vi "FacadeResizable1DArray(I32).vi"(0 "Data In":T4, 2 "Display State In":T2, 3 "Container State":T3) -> (6 "Data Out":T4, 7 "Display State Out":T2, 8 "Action":T1)   [LabVIEW 2011, in "Resizable1DArray(I32).xctl"]
uses:
  <vilib>/_probes/SAPHIR/ViBox - Probes/Resizable1DArray/Resizable1DArray(I32)/Resizable1DArray(I32).xctl
  <vilib>/_probes/SAPHIR/ViBox - Probes/Resizable1DArray/Resizable1DArray(I32)/DataResizable1DArray(I32).ctl
  <vilib>/_xctls/Container State.ctl
  <vilib>/_probes/SAPHIR/ViBox - Probes/Resizable1DArray/Resizable1DArray(I32)/StateResizable1DArray(I32).ctl
  <vilib>/_xctls/Action.ctl
  <vilib>/_xctls/XControlSupport.lvlib
panel:
  in  "Format":string caption="Format :"
  out "Numeric":i32
  out "[I32]":i32[](array[numeric])
  # "Display Options"
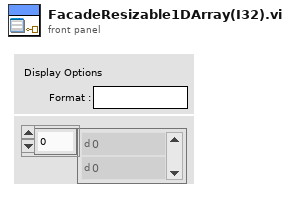
[diagram p1: front panel]
types:
  T1 = typedef "XControlSupport.lvlib/Action.ctl" = cluster{"Data Changed?":bool, "State Changed?":bool, "Action Name":string}
  T2 = typedef "Resizable1DArray(I32).xctl/StateResizable1DArray(I32).ctl" = cluster{"Height":u32}
  T3 = typedef "XControlSupport.lvlib/Container State.ctl" = cluster{"Indicator?":bool, "Run Mode?":bool, " Refnum":refnum<vi>}
  T4 = typedef "Resizable1DArray(I32).xctl/DataResizable1DArray(I32).ctl" = i32[]
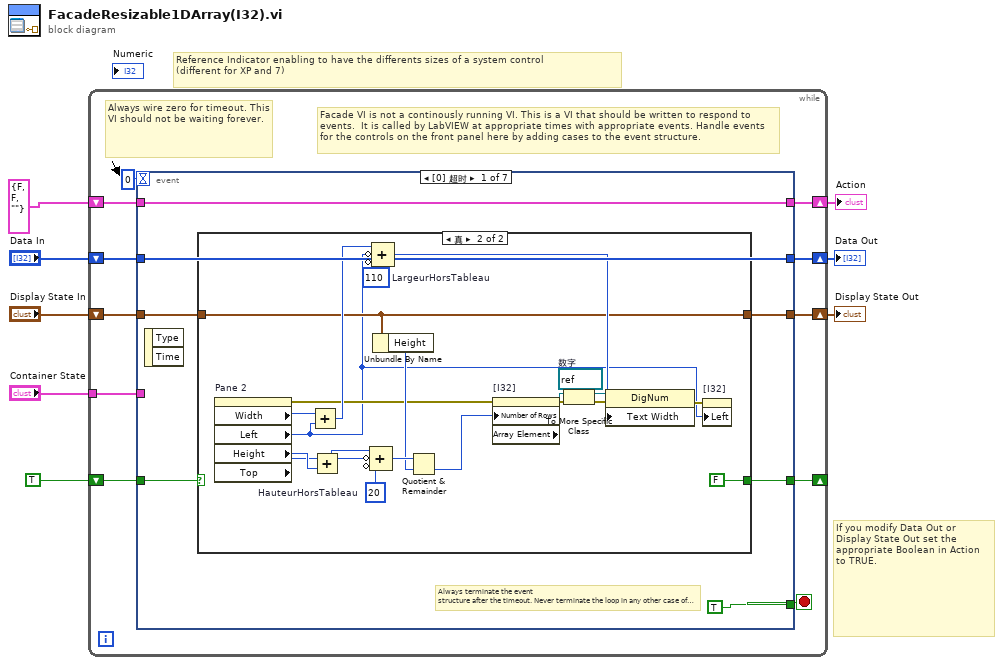
[diagram p0: block diagram]
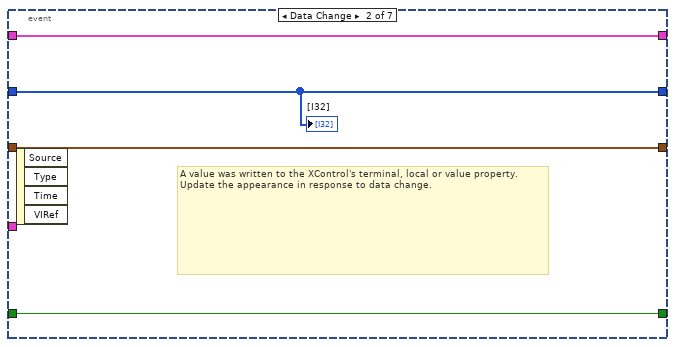
[diagram p3: hidden frame]
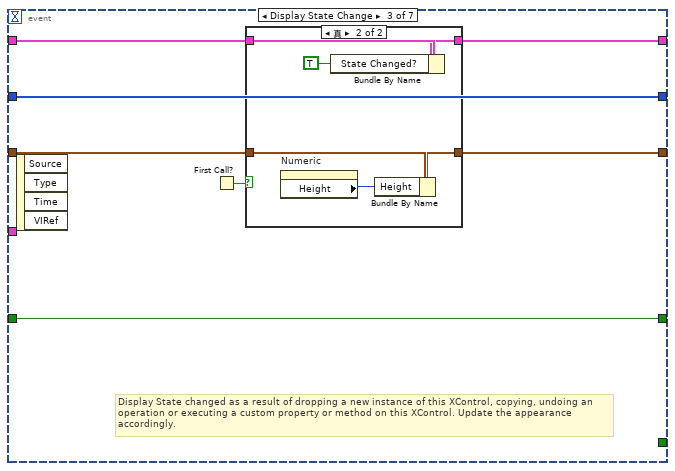
[diagram p4: hidden frame]
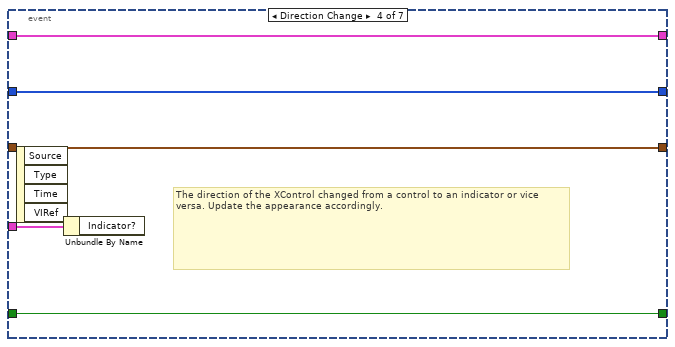
[diagram p6: hidden frame]
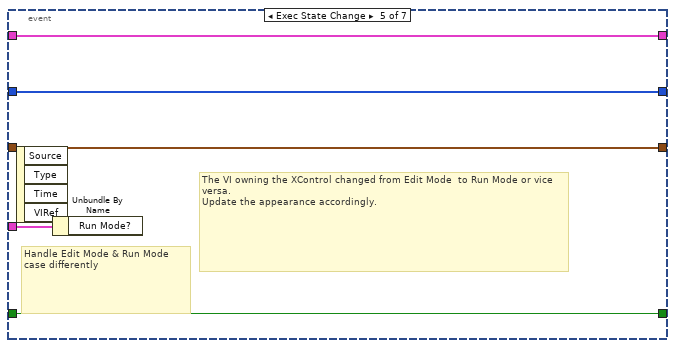
[diagram p7: hidden frame]
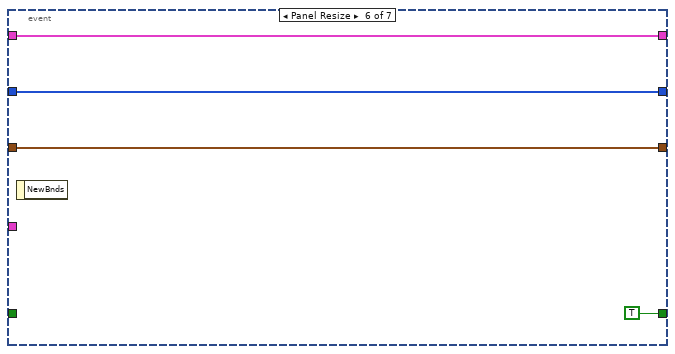
[diagram p8: hidden frame]
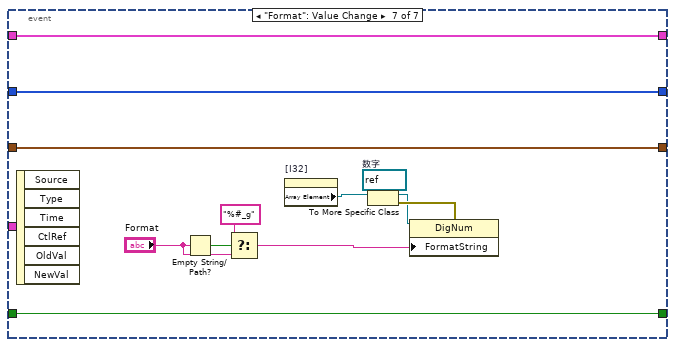
[diagram p9: hidden frame]
diagram:
  # "Reference Indicator enabling to have the differents sizes of a system control\n(different for XP and 7)"
  # "If you modify Data Out or\nDisplay State Out set the\nappropriate Boolean in Action\nto TRUE."
  n1 = while {
    shift-right: [w18] -> w6
    shift-left: "Display State In" -> [w19]
    tunnel: "Container State" -> [w15]
    shift-right: [w13] -> w8
    shift-left: "Data In" -> [w14]
    shift-right: [w11] -> w4
    shift-left: T1 {"Data Changed?"=FALSE, "State Changed?"=FALSE, "Action Name"=""} ("Action") -> [w12]
    shift-right: [w9] -> _
    shift-left: TRUE -> [w10]
    stop <- w17 stop-if-true
    # "Facade VI is not a continously running VI. This is a VI that should be written to respond to events.  It is called by LabVIEW at appropriate times with appropriate events. Handle events for the controls on the front panel here by adding cases to the event structure."
    # "Always wire zero for timeout. This\nVI should not be waiting forever."
    n2 = event shown="[0] 超时" {
      selector: _ -> [_ _ _ _ _ _ _]
      dyn-events: _ -> [_ _ _ _ _ _ _]
      timeout: 0 -> [_ _ _ _ _ _ _]
      tunnel: w19 -> [w21 w53 w55 w72 w77 w81 w91]
      tunnel: [w20 w53 w54 w72 w77 w81 w91] -> w18
      tunnel: [TRUE _ _ _ _ _ _] -> w17
      tunnel: w15 -> [_ _ _ w73 w78 _ _]
      tunnel: w14 -> [w24 w51 w60 w71 w76 w82 w92]
      tunnel: [w24 w51 w60 w71 w76 w82 w92] -> w13
      tunnel: [w25 w52 w56 w70 w75 w80 w93] -> w11
      tunnel: w12 -> [w25 w52 w57 w70 w75 w80 w93]
      tunnel: w10 -> [w23 w50 w59 w69 w74 _ w94]
      tunnel: [w22 w50 w59 w69 w74 TRUE w94] -> w9
      event Timeout {
        # "Always terminate the event\nstructure after the timeout. Never terminate the loop in any other case of the event structure."
        n3 = event-data() -> ()  [unwired: 3 out]
        n4 = case shown="真" w23 {
          selector: w23 -> [w28 _]
          tunnel: [w28 FALSE] -> w22
          tunnel: w21 -> [w27 w36]
          tunnel: [w27 w36] -> w20
          frame False {
          }
          frame True {
            w42 = refnum<vi> refnum  # 数字
            w40 = i16 20  # HauteurHorsTableau
            w41 = i16 110  # LargeurHorsTableau
            n5 = property on="Pane 2" class="Pane"() -> (error out=w32:errorcluster, "Width"=w33:u32, "Left"=w31:i32, "Height"=w30:u32, "Top"=w29:i32)  [unwired: 2 in, 1 out]
            n6 = Add(x=w33, y=w31) -> (x+y=w39:u32)
            n7 = Add(x=w29, y=w30) -> (x+y=w49:u32)
            n8 = Compound Arithmetic op=ADD(w49, invert w29, invert w40) -> (w45:u32)
            n9 = Compound Arithmetic op=ADD(w39, invert w31, invert w41) -> (w38:u32)
            n10 = Unbundle By Name(w36) -> ("Height"=w35:u32)
            n11 = Quotient & Remainder(x=w45, y=w35) -> (floor(x/y)=w34:u32)  [unwired: 1 out]
            n12 = property on="[I32]" class="Arr (严格)"(error in=w32, "Number of Rows"=w34) -> (error out=w46:errorcluster, "Array Element"=w44:refnum<vi>)  [unwired: 1 in, 1 out]
            n13 = To More Specific Class(target class=w42, reference=w44, error in=w46) -> (specific class reference=w43:refnum<vi>, error out=w47:errorcluster)
            n14 = property class="DigNum"(reference=w43, error in=w47, "Text Width"=w38) -> (error out=w48:errorcluster)  [unwired: 1 out]
            n15 = property on="[I32]" class="Arr (严格)"(error in=w48, "Left"=w31) -> ()  [unwired: 1 in, 2 out]
          }
        }
      }
      event Data Change {
        # "A value was written to the XControl's terminal, local or value property.\nUpdate the appearance in response to data change."
        n16 = event-data() -> ()  [unwired: 5 out]
        "[I32]" <- w51
      }
      event Display State Change {
        # "Display State changed as a result of dropping a new instance of this XControl, copying, undoing an operation or executing a custom property or method on this XControl. Update the appearance accordingly."
        n17 = event-data() -> ()  [unwired: 5 out]
        n18 = First Call?() -> (First Call?: T/F=w58:bool)
        n19 = case shown="真" w58 {
          tunnel: w55 -> [w62 w68]
          tunnel: [w62 w67] -> w54
          tunnel: w57 -> [w61 w65]
          tunnel: [w61 w64] -> w56
          frame False {
          }
          frame True {
            n20 = property on="Numeric" class="DigNum (严格)"() -> ("Height"=w66:u32)  [unwired: 2 in, 2 out]
            n21 = Bundle By Name(cluster=w65, "State Changed?"=TRUE) -> (w64:T1)
            n22 = Bundle By Name(cluster=w68, "Height"=w66) -> (w67:T2)
          }
        }
      }
      event Direction Change {
        # "The direction of the XControl changed from a control to an indicator or vice versa. Update the appearance accordingly."
        n23 = event-data() -> ()  [unwired: 5 out]
        n24 = Unbundle By Name(w73) -> ()  [unwired: 1 out]
      }
      event Exec State Change {
        # "The VI owning the XControl changed from Edit Mode  to Run Mode or vice versa.\nUpdate the appearance accordingly."
        # "Handle Edit Mode & Run Mode\ncase differently"
        n25 = event-data() -> ()  [unwired: 5 out]
        n26 = Unbundle By Name(w78) -> ()  [unwired: 1 out]
      }
      event Panel Resize {
        n27 = event-data() -> ()  [unwired: 2 out]
      }
      event "Format": Value Change {
        w84 = refnum<vi> refnum  # 数字
        n28 = event-data() -> ()  [unwired: 7 out]
        n29 = Empty String/Path?(string/path="Format") -> (empty?=w88:bool)
        n30 = Select(t="%#_g", s=w88, f="Format") -> (s? t:f=w90:string)
        n31 = property on="[I32]" class="Arr (严格)"() -> ("Array Element"=w87:refnum<vi>)  [unwired: 2 in, 2 out]
        n32 = To More Specific Class(target class=w84, reference=w87) -> (specific class reference=w85:refnum<vi>, error out=w86:errorcluster)  [unwired: 1 in]
        n33 = property class="DigNum"(reference=w85, error in=w86, "FormatString"=w90) -> ()  [unwired: 2 out]
      }
    }
  }
  "Display State Out" <- w6
  "Data Out" <- w8
  "Action" <- w4
